vi "Set Master Node Analog Out.vi"(8 "error in (no error)":errorcluster, 9 "idxMaster":i32, 10 "idxChannel":i32, 11 "hdwf":i32) -> (0 "error out":errorcluster, 3 "hdwf out":i32)   [LabVIEW 2012, in "AnalogDiscSDKLv.lvlib"]
doc: "extern \"C\" __declspec(dllexport) int SetMasterNode_AnalogOut(\n HDWF hdwf,\n int idxChannel,\n int idxMaster\n );"
uses:
  <instrlib>/AnalogDiscSDKLv/AnalogDiscSDKLv.lvlib
  <instrlib>/AnalogDiscSDKLv/AnalogDiscSDKLv.dll
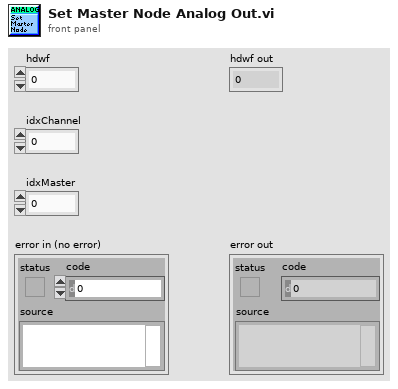
[diagram p1: front panel]
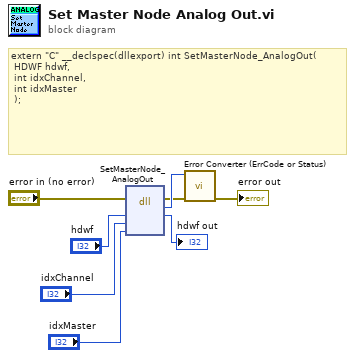
[diagram p0: block diagram]
diagram:
  # "extern \"C\" __declspec(dllexport) int SetMasterNode_AnalogOut(\n\tHDWF hdwf,\n\tint idxChannel,\n\tint idxMaster\n\t);"
  n1 = dll-call lib="C:/Program Files (x86)/National Instruments/LabVIEW 2012/instr.lib/AnalogDiscSDKLv/AnalogDiscSDKLv.*" fn="SetMasterNode_AnalogOut"(error in="error in (no error)", "hdwf"="hdwf", "idxChannel"="idxChannel", "idxMaster"="idxMaster") -> (error out=w2:errorcluster, w3:i32, "hdwf"=→"hdwf out":i32)  [unwired: 4 in, 1 out]
  n2 = call <instrlib>:"Error Converter (ErrCode or Status).vi"("error in (no error)"=w2, "error code"=w3) -> ("error out"=→"error out":errorcluster)  [unwired: 9 in]
